vi "ArrayRead_I.vi"(0 "Current (or Cued Trial Parameters)":i32[](array[numeric])) -> (4 "Value 0":i32, 6 "Value 1":i32, 8 "Value 2":i32, 10 "Value 3":i32, 11 "Value 8":i32, 12 "Value 7":i32, 13 "Value 6":i32, 14 "Value 5":i32, 15 "Value 4":i32)   [LabVIEW 2009]
doc: "This VI allows you to access the first 9 elements in a double array. If there are less elements, you will get the default value of zero in return."
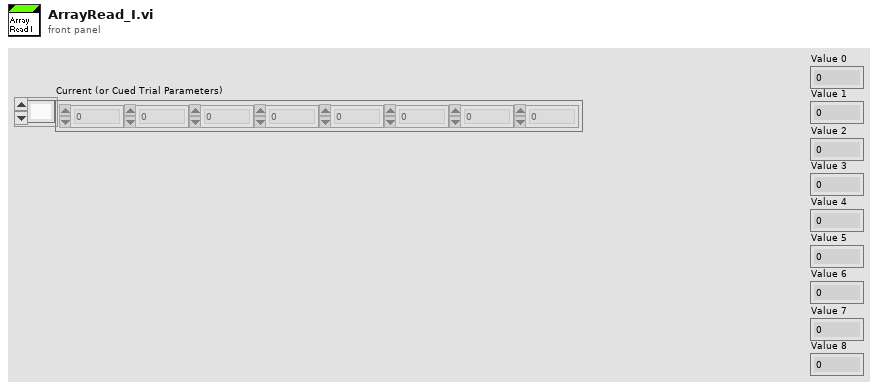
[diagram p1: front panel]
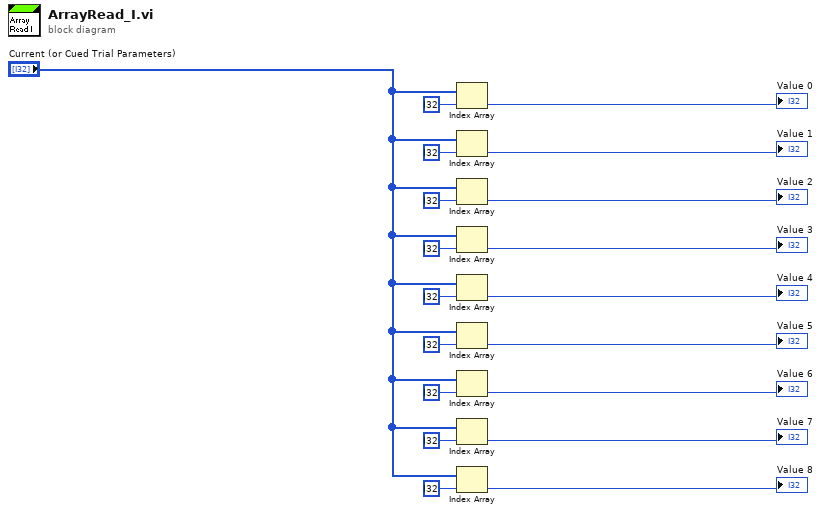
[diagram p0: block diagram]
diagram:
  n1 = Index Array(array="Current (or Cued Trial Parameters)", index=i32 ?) -> (element=→"Value 0":i32)
  n2 = Index Array(array="Current (or Cued Trial Parameters)", index=i32 ?) -> (element=→"Value 1":i32)
  n3 = Index Array(array="Current (or Cued Trial Parameters)", index=i32 ?) -> (element=→"Value 2":i32)
  n4 = Index Array(array="Current (or Cued Trial Parameters)", index=i32 ?) -> (element=→"Value 3":i32)
  n5 = Index Array(array="Current (or Cued Trial Parameters)", index=i32 ?) -> (element=→"Value 4":i32)
  n6 = Index Array(array="Current (or Cued Trial Parameters)", index=i32 ?) -> (element=→"Value 5":i32)
  n7 = Index Array(array="Current (or Cued Trial Parameters)", index=i32 ?) -> (element=→"Value 6":i32)
  n8 = Index Array(array="Current (or Cued Trial Parameters)", index=i32 ?) -> (element=→"Value 7":i32)
  n9 = Index Array(array="Current (or Cued Trial Parameters)", index=i32 ?) -> (element=→"Value 8":i32)
